vi "fmt_createFormatBuffer.vi"(0 "rows":i32=1, 1 "max rows":i32=1048576, 2 "start time":timestamp, 5 "columns":T1, 7 "time column mode":T4, 9 "predifed formatted value length":i32=20, 11 "error in (no error)":errorcluster, 12 "start row":i32, 13 "max styles":i32) -> (4 "Format buffers out":T5, 15 "error out":errorcluster)   [LabVIEW 2020, in "NI_ExcelFile.lvlib"]
uses:
  <vilib>/express/express shared/NI_ExcelFile/NI_ExcelFile.lvlib
  <vilib>/express/express shared/NI_ExcelFile/Ctrls/fmt_formatBuffer.ctl
  <vilib>/express/express shared/NI_ExcelFile/Ctrls/TimeColumnMode.ctl
  <vilib>/express/express shared/NI_ExcelFile/Ctrls/Columns.ctl
  <vilib>/express/express shared/NI_ExcelFile/Ctrls/ColumnInfo.ctl
  <vilib>/express/express shared/NI_ExcelFile/Ctrls/DataType.ctl
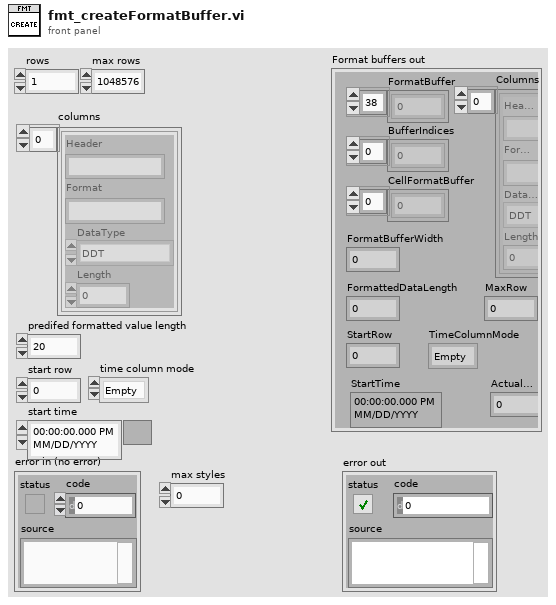
[diagram p1: front panel]
types:
  T1 = typedef "NI_ExcelFile.lvlib/Columns.ctl" = T2[]
  T2 = typedef "NI_ExcelFile.lvlib/ColumnInfo.ctl" = cluster{"Header":string, "Format":string, "DataType":T3, "Length":u64}
  T3 = typedef "NI_ExcelFile.lvlib/DataType.ctl" = enum16{"DDT", "WFM", "Array of STR", "Array of DBL", "Array of I8", "Array of I16", "Array of I32", "Array of I64", "Array of SGL", "Array of U8", "Array of U16", "Array of U32", "Array of U64", "Array of Time"}
  T4 = typedef "NI_ExcelFile.lvlib/TimeColumnMode.ctl" = enum16{"Empty", "OnePerCh", "One"}
  T5 = typedef "NI_ExcelFile.lvlib/fmt_formatBuffer.ctl" = cluster{"FormatBuffer":u8[], "BufferIndices":i32[], "CellFormatBuffer":u8[], "FormatBufferWidth":i32, "FormattedDataLength":i32, "MaxRow":i32, "StartRow":i32, "TimeColumnMode":T4, "StartTime":timestamp, "Columns":T1, "ActualLength":i32}
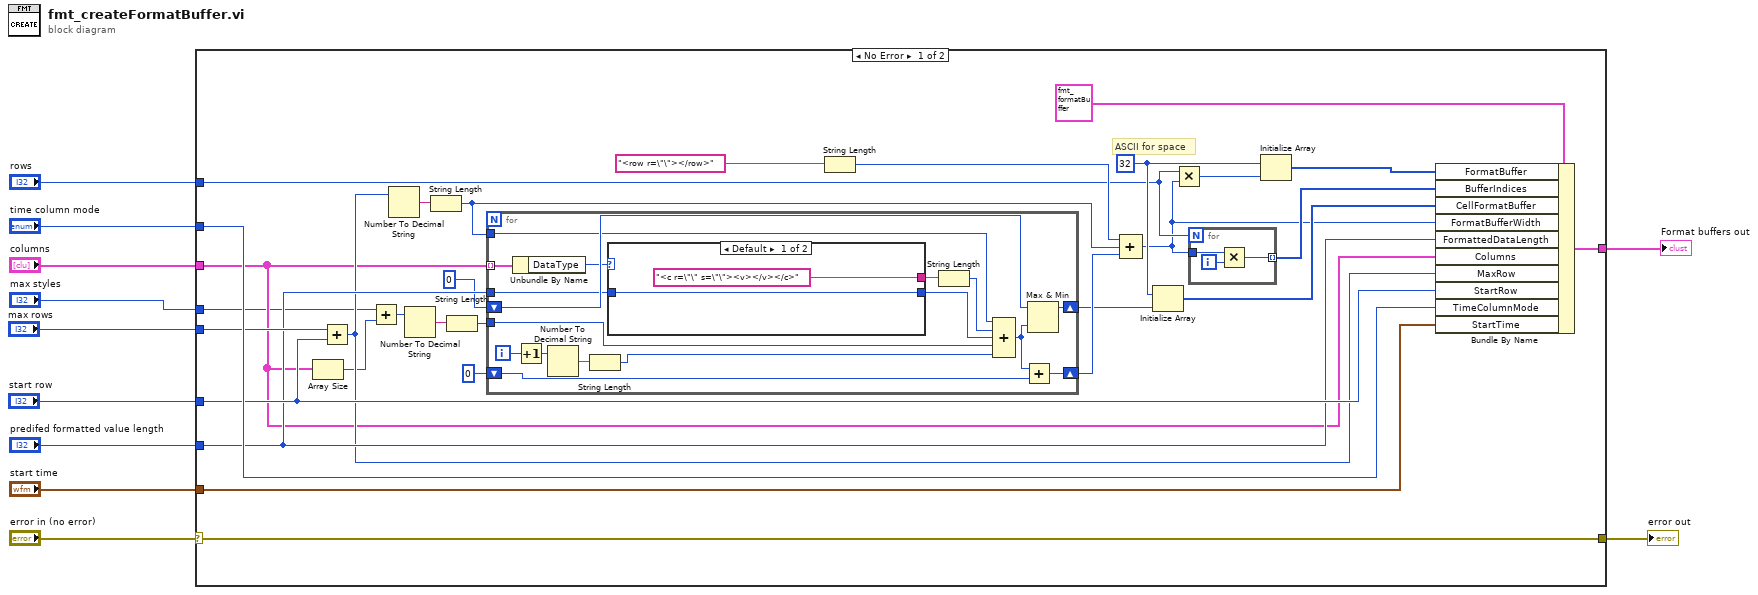
[diagram p0: block diagram]
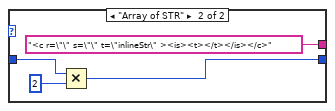
[diagram p2: hidden frame]
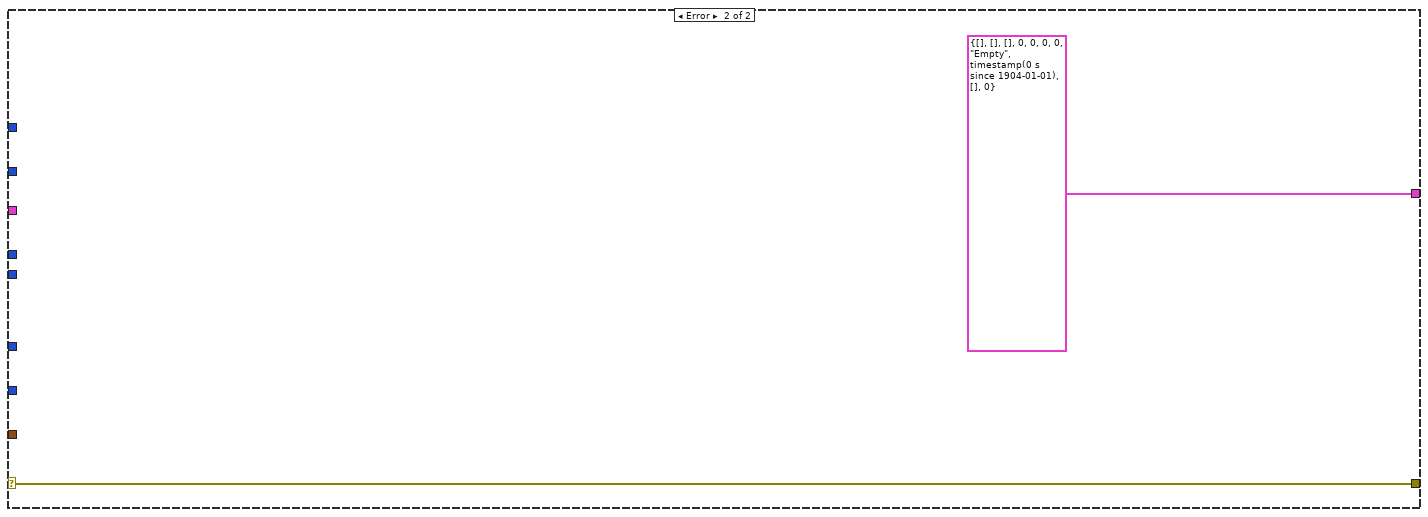
[diagram p3: hidden frame]
diagram:
  n1 = case shown="No Error" "error in (no error)" {
    selector: "error in (no error)" -> [w28 w69]
    tunnel: [w33 T5 {"FormatBuffer"=[], "BufferIndices"=[], "CellFormatBuffer"=[], "FormatBufferWidth"=0, "FormattedDataLength"=0, "MaxRow"=0, "StartRow"=0, "TimeColumnMode"=enum."Empty", "StartTime"=timestamp(0 s since 1904-01-01), "Columns"=[], "ActualLength"=0} ("Format buffers")] -> w11
    tunnel: "rows" -> [w31 _]
    tunnel: "predifed formatted value length" -> [w24 _]
    tunnel: "start row" -> [w27 _]
    tunnel: "time column mode" -> [w29 _]
    tunnel: [w28 w69] -> w6
    tunnel: "max rows" -> [w26 _]
    tunnel: "start time" -> [w25 _]
    tunnel: "columns" -> [w15 _]
    tunnel: "max styles" -> [w14 _]
    frame No Error {
      w37 = u8 32 ("element")
      # "ASCII for space"
      n2 = Array Size(array=w15) -> (size(s)=w12:i32)
      n3 = Add(x=w26, y=w27) -> (x+y=w20:i32)
      n4 = Add(x=w14, y=w12) -> (x+y=w13:i32)
      n5 = Number To Decimal String(number=w20) -> (decimal integer string=w40:string)  [unwired: 1 in]
      n6 = Number To Decimal String(number=w13) -> (decimal integer string=w19:string)  [unwired: 1 in]
      n7 = String Length(string=w40) -> (length=w22:i32)
      n8 = String Length(string=w19) -> (length=w18:i32)
      n9 = for {
        tunnel: w15 -> [w57] mode=indexing
        tunnel: w24 -> [w55]
        shift-right: [w43] -> w21
        shift-left: 0 -> [w42]
        tunnel: w22 -> [w50]
        tunnel: w18 -> [w47]
        shift-right: [w46] -> w17
        shift-left: 0 -> [w58]
        i -> [w54]
        n10 = Unbundle By Name(w57) -> ("DataType"=w56:T3)
        n11 = Increment(x=w54) -> (x+1=w53:i32)
        n12 = Number To Decimal String(number=w53) -> (decimal integer string=w52:string)  [unwired: 1 in]
        n13 = String Length(string=w52) -> (length=w45:i32)
        n14 = case shown="Default" w56 {
          tunnel: w55 -> [w60 w64]
          tunnel: [w60 w62] -> w48
          tunnel: ["<c r=\"\" s=\"\"><v></v></c>" "<c r=\"\" s=\"\" t=\"inlineStr\" ><is><t></t></is></c>"] -> w51
          frame Default {
          }
          frame "Array of STR" {
            n15 = Multiply(x=w64, y=2) -> (x*y=w62:i32)
          }
        }
        n16 = String Length(string=w51) -> (length=w49:i32)
        n17 = Compound Arithmetic op=ADD(w50, w49, w48, w47, w45) -> (w44:i32)
        n18 = Add(x=w44, y=w42) -> (x+y=w43:i32)
        n19 = Max & Min(x=w58, y=w44) -> (max(x,y)=w46:i32)  [unwired: 1 out]
      }
      n20 = String Length(string="<row r=\"\"></row>") -> (length=w38:i32)
      n21 = Compound Arithmetic op=ADD(w38, w22, w21) -> (w30:i32)
      n22 = Initialize Array(w37, w17) -> (w36:u8[])
      n23 = Multiply(x=w31, y=w30) -> (x*y=w39:i32)
      n24 = for {
        N: w31 -> [_]
        tunnel: w30 -> [w67]
        tunnel: [w65] -> w32 mode=indexing
        i -> [w66]
        n25 = Multiply(x=w67, y=w66) -> (x*y=w65:i32)
      }
      n26 = Initialize Array(w37, w39) -> (w35:u8[])
      n27 = Bundle By Name(cluster=T5 {"FormatBuffer"=[], "BufferIndices"=[], "CellFormatBuffer"=[], "FormatBufferWidth"=0, "FormattedDataLength"=0, "MaxRow"=0, "StartRow"=0, "TimeColumnMode"=enum."Empty", "StartTime"=timestamp(0 s since 1904-01-01), "Columns"=[], "ActualLength"=0} ("Format buffers"), "FormatBuffer"=w35, "BufferIndices"=w32, "CellFormatBuffer"=w36, "FormatBufferWidth"=w30, "FormattedDataLength"=w24, "Columns"=w15, "MaxRow"=w20, "StartRow"=w27, "TimeColumnMode"=w29, "StartTime"=w25) -> (w33:T5)
    }
    frame Error {
    }
  }
  "Format buffers out" <- w11
  "error out" <- w6
